vi "BPE Boiling Point Elavation of Saline Water(Centigrade Degree).vi"(1 "Salinity":dbl, 2 "Sailne Water Temprature":dbl[unit]) -> (0 "BPE":dbl[unit])   [LabVIEW 2018]
panel:
  out "BPE":dbl[unit](slide) scale=0.0..100.0
  out "Saline Water Temprature":dbl[unit](slide) scale=0.0..100.0
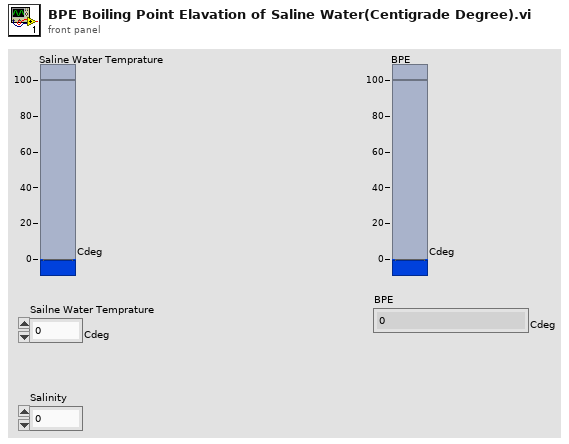
[diagram p1: front panel]
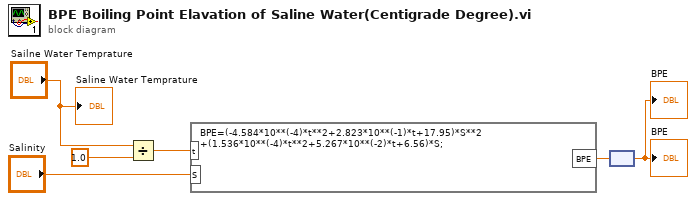
[diagram p0: block diagram]
diagram:
  n1 = Divide(x="Sailne Water Temprature", y=dbl[unit] 1.0) -> (x/y=w6:dbl)
  n2 = formula code="BPE=(-4.584*10**(-4)*t**2+2.823*10**(-1)*t+17.95)*S**2\n+(1.536*10**(-4)*t**2+5.267*10**(-2)*t+6.56)*S;"("t"=w6, "S"="Salinity") -> ("BPE"=w2:dbl)
  n3 = node(w2) -> (→"BPE" →"BPE":dbl[unit])
  "Saline Water Temprature" <- "Sailne Water Temprature"
